vi "Intrinsic Imager.vi"() -> ()   [LabVIEW 2016]
uses:
  <vilib>/vision/Image Controls.llb/IMAQ Image.ctl
  <vilib>/userdefined/High Color/IMAQdx.ctl
  <instrlib>/niHWS/nihws.llb/niHWS Open File Permissions ID.ctl
  <vilib>/Utility/error.llb/DialogType.ctl
  <vilib>/DAQmx/read.llb/DAQmx Read (Analog Wfm 1Chan NSamp).vi
  <vilib>/Analysis/baseanly.llb/Mean (DBL).vi
  <instrlib>/niHWS/nihws.llb/niHWS Write Analog DBL.vi
  <vilib>/DAQmx/miscellaneous.llb/DAQmx Fill In Error Info.vi
  <instrlib>/niHWS/nihws.llb/niHWS Write Analog WDT.vi
  <instrlib>/niHWS/nihws.llb/niHWS Write Digital 2D U16.vi
  <vilib>/vision/NI_Vision_Development_Module.lvlib
  <resource>/objmgr/daqmx.rc
  <vilib>/Analysis/NI_AALBase.lvlib
  <vilib>/vision/driver/NI_Vision_Acquisition_Software.lvlib
panel:
  in  "Single trial":bool
  in  "Analysis":enum32{"Amp", "Angle", "Amp/Angle"}(radio)
  in  "Analyze":bool
  in  "Period (ms)":dbl=16641.0
  in  "Pixel Thr":dbl=4095.0
  in  "Magnify":bool
  in  "PseudoColor":bool
  out "Frames":u32 caption="Image Number"
  out "Rep. Fps":dbl caption="Frame Rate"
  out "Fps":dbl
  out "Ephys Rate":dbl=1000.0
  in  "Final res.":dbl=512.0
  out "Image Parameters : Bits per Pixel":u32
  out "Numeric":i32
  out "Setup":i32
  out "PPhocus?":bool
  out "file handle out":u32
  out "Recording":bool
  in  "stop":bool
  out "Raw Image":T1(plugin-control)
  out "Rec Time":dbl
  out "Photodiode display":waveform(dbl)(graph)
  in  "Recording Path":path
  in  "Rec":bool
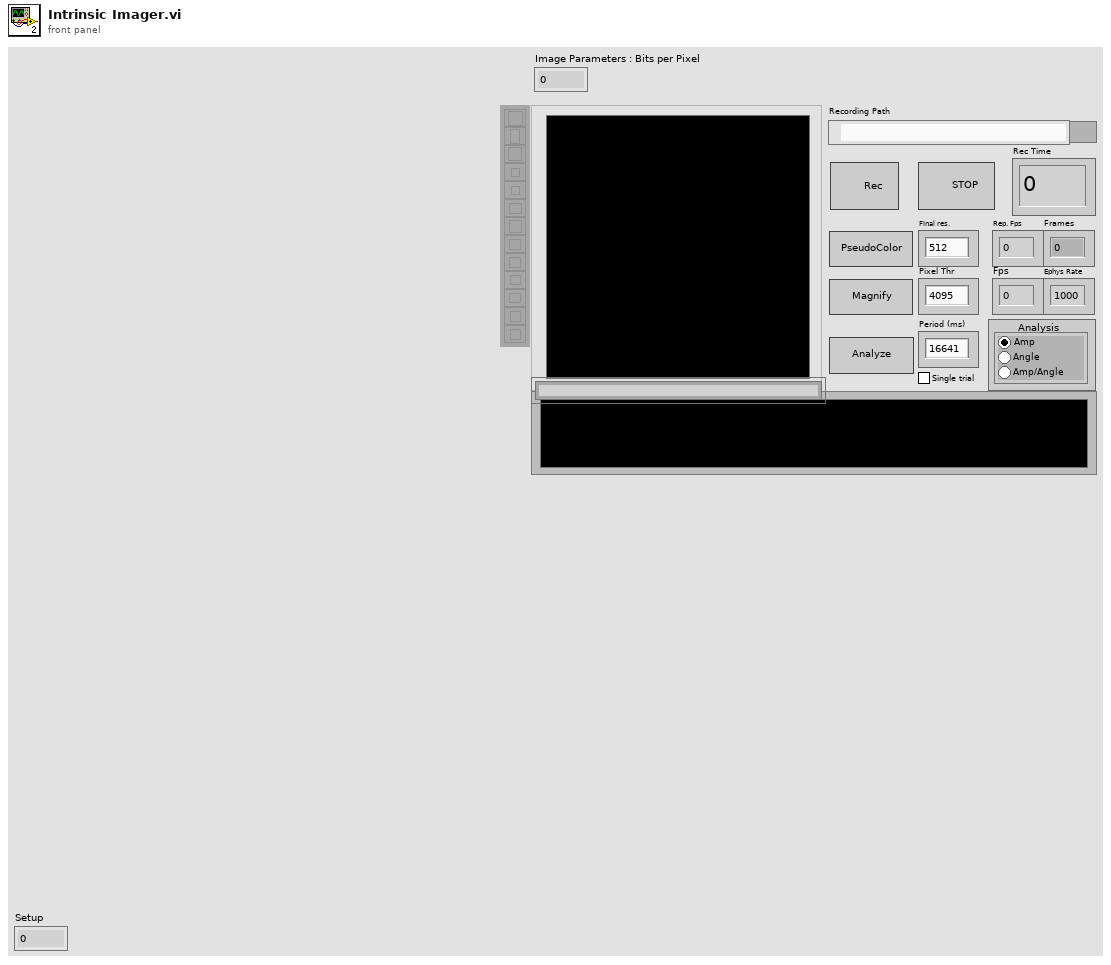
[diagram p1: front panel]
types:
  T1 = typedef "IMAQ Image.ctl" = refnum<image>
  T2 = typedef "IMAQdx.ctl" = refnum<k21>
  T3 = typedef "Image Type" = u32
  T4 = cluster{"IMAQ Session Out":refnum<k11>, "OriginalImage":T1, "error out":errorcluster, "size":cluster{dbl, i32}[], "Cropped Image":T1, "IMAQdx Session":T2, "Camera":string, "Image Type":T3, "Mirrored Image":T1, "Rotated Image":T1}
  T5 = typedef "niHWS Open File Permissions ID.ctl" = enum32{"Read Only", "Read/Write Existing", "Read/Write/Create New", "Read/Write/Create New Always"}
  T6 = enum32{"Average", "Min", "Max", "Clear  if < ", "Clear  if < or =", "Clear  if =", "Clear  if > or =", "Clear  if >"}
  T7 = enum32{"Invalid", "Standard", "Closed", "Hidden", "Minimized", "Maximized"}
  T8 = cluster{"Interpolation Type":enum32{"Zero Order", "Bilinear", "Quadratic", "Cubic", "Bilinear Fixed"}, "Destination Width":u32, "Destination Height":u32, "Fill Value":sgl}
  T9 = cluster{"Type":u32, "Version":u32, "Flags":u32, "SerialNumberHigh":u32, "SerialNumberLow":u32, "BusType":u32, "InterfaceName":string, "VendorName":string, "ModelName":string, "CameraFileName":string, "CameraAttributeURL":string}[]
  T10 = cluster{"Type":u32, "Version":u32, "Flags":u32, "SerialNumberHigh":u32, "SerialNumberLow":u32, "BusType":u32, "InterfaceName":string, "VendorName":string, "ModelName":string, "CameraFileName":string, "CameraAttributeURL":string}
  T11 = typedef "DialogType.ctl" = u16
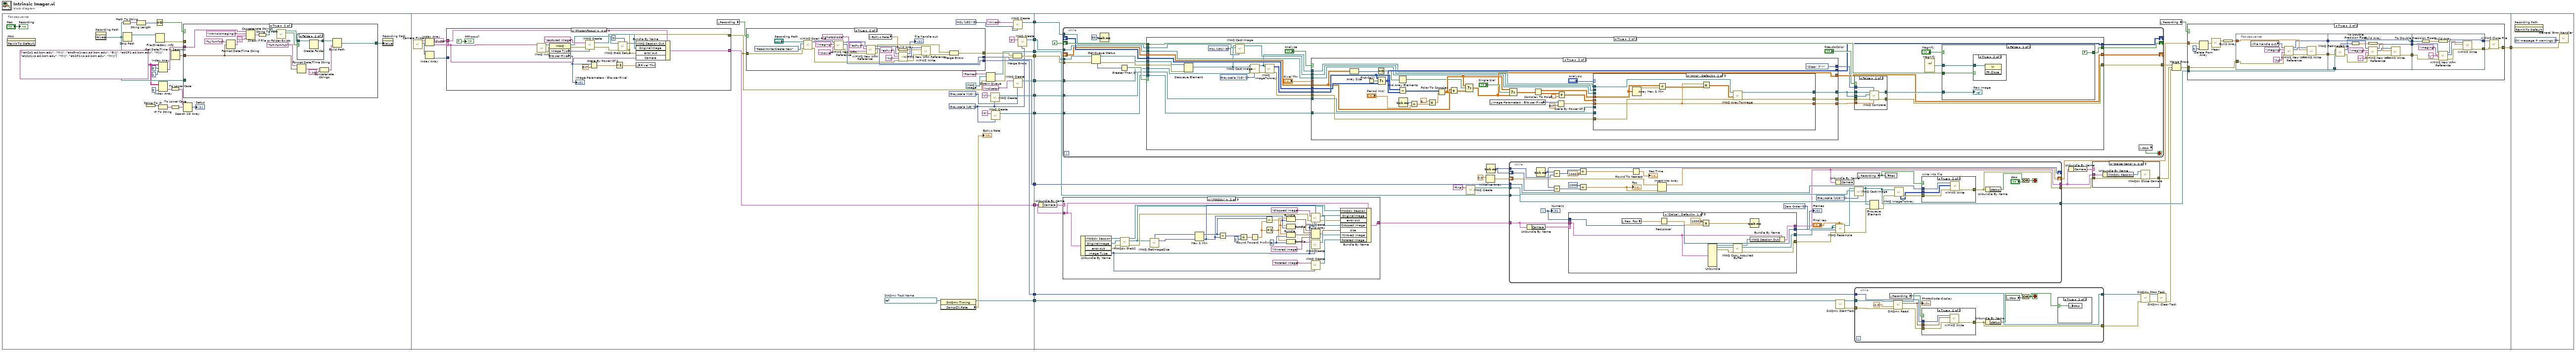
[diagram p0: block diagram]
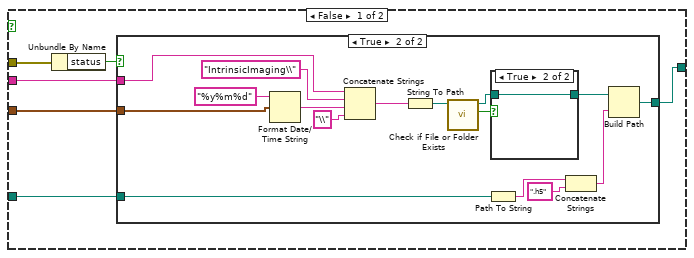
[diagram p2: hidden frame]
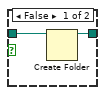
[diagram p4: hidden frame]
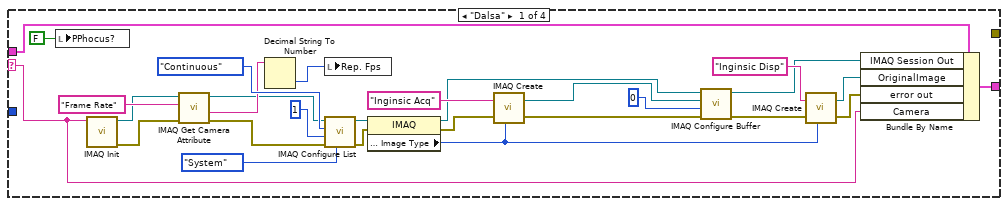
[diagram p6: hidden frame]
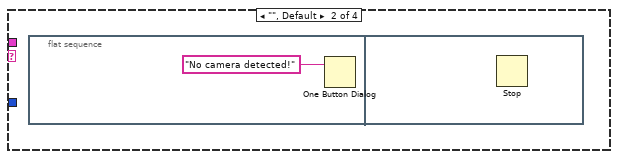
[diagram p7: hidden frame]
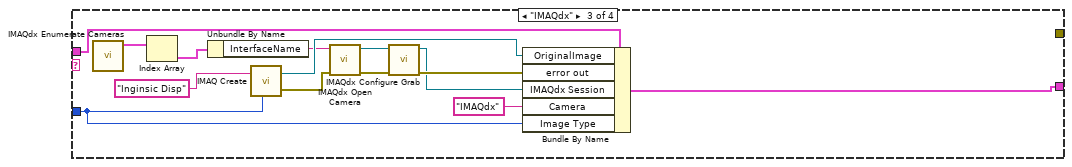
[diagram p8: hidden frame]
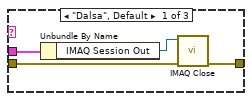
[diagram p10: hidden frame]
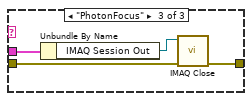
[diagram p11: hidden frame]
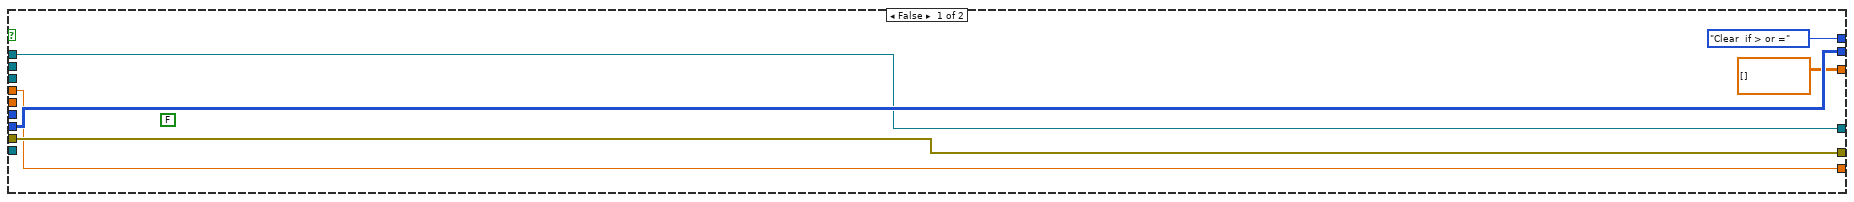
[diagram p13: hidden frame]
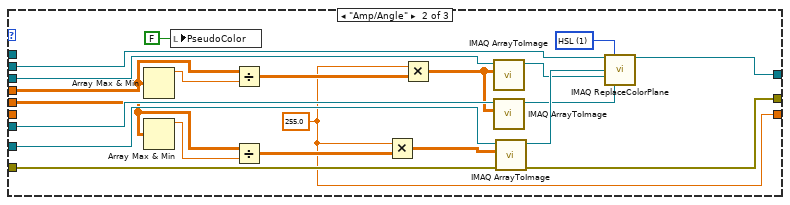
[diagram p14: hidden frame]
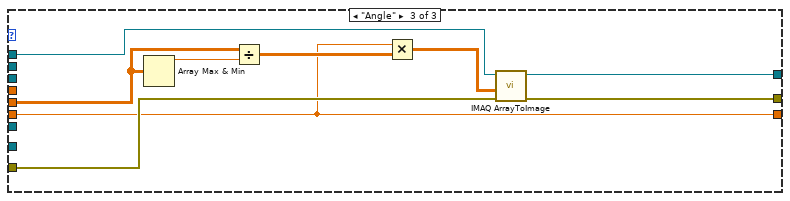
[diagram p15: hidden frame]
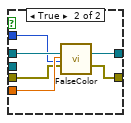
[diagram p16: hidden frame]
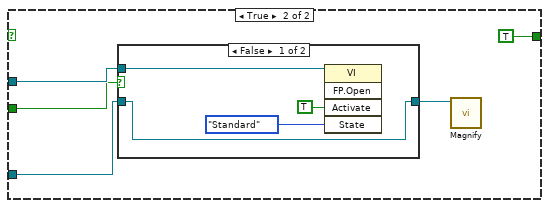
[diagram p18: hidden frame]
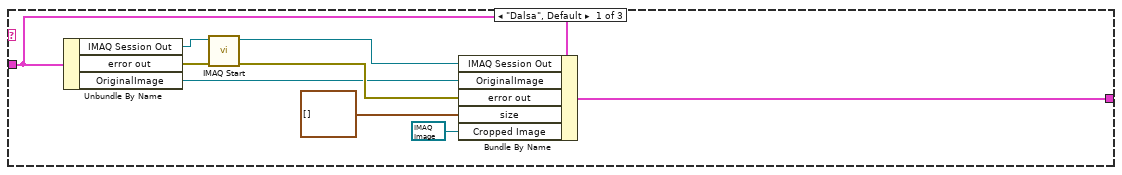
[diagram p20: hidden frame]
diagram:
  n1 = flat-sequence {
    tunnel: [w109] -> w12
    tunnel: [w108] -> w11
    tunnel: [w104] -> w9
    tunnel: [w96] -> w8
    tunnel: [w95] -> w7
    tunnel: [w92] -> w6
    tunnel: [w90] -> w5
    tunnel: [w88] -> w4
    tunnel: [w87] -> w3
    tunnel: [w83] -> w2
    tunnel: [w80] -> w1
    tunnel: w12 -> [w225]
    tunnel: w11 -> [w226]
    tunnel: [w224] -> w10
    tunnel: w9 -> [w211]
    tunnel: w8 -> [w208]
    tunnel: w7 -> [w209]
    tunnel: w6 -> [w206]
    tunnel: w5 -> [w205]
    tunnel: w4 -> [w204]
    tunnel: w3 -> [w203]
    tunnel: w2 -> [w202]
    tunnel: w1 -> [w201]
    tunnel: w10 -> [w637]
    frame #0 {
      w19 = string[][] [["at-2p1.ad.bcm.edu", "M:\\"], ["at-s5no1new.ad.bcm.edu", "E:\\"], ["at-2P1.ad.bcm.edu", "M:\\"], ["at-2p1xp.ad.bcm.edu", "M:\\"], ["at-2P1xp.ad.bcm.edu", "M:\\"]]
      n2 = invoke on="stop" class="Bool (strict)" method="Reinit To Default"() -> ()  [unwired: 3 in, 3 out]
      n3 = property on="Recording Path" class="Path"() -> ("Value"=w26:path)  [unwired: 2 in, 2 out]
      n4 = Path To String(path=w26) -> (string=w31:string)
      n5 = Strip Path(path=w26) -> (stripped path=w25:path)  [unwired: 1 out]
      n6 = String Length(string=w31) -> (length=w30:i32)
      n7 = String To IP() -> (0:w23:u32)  [unwired: 1 in]
      n8 = Equal To 0?(x=w30) -> (x = 0?=w29:bool)
      n9 = File/Directory Info(path=w25) -> (error out=w24:errorcluster)  [unwired: 1 in, 6 out]
      n10 = IP To String(2:w23) -> (0:w15:string)  [unwired: 1 in]
      n11 = Index Array(array=w19, index (row)=0 ("disabled index (row)"), index (col)=1 ("disabled index (col)")) -> (element=w18:string)
      n12 = Index Array(array=w19, index (col)=0 ("disabled index (col)")) -> (element=w17:string[])  [unwired: 1 in]
      n13 = To Lower Case(string=w17) -> (all lower case string=w16:string[])
      n14 = To Lower Case(string=w15) -> (all lower case string=w14:string)
      n15 = Get Date/Time In Seconds() -> (seconds since 1Jan1904=w32:timestamp)
      n16 = case shown="True" w29 {
        tunnel: w32 -> [w36 w65]
        tunnel: w26 -> [w37 _]
        tunnel: [w38 w63] -> w28
        tunnel: w24 -> [w34 _]
        tunnel: w18 -> [w33 w59]
        frame False {
          n17 = Unbundle By Name(w34) -> ("status"=w35:bool)
          n18 = case shown="True" w35 {
            tunnel: [w39 w46] -> w38
            tunnel: w37 -> [w39 w45]
            tunnel: w36 -> [_ w41]
            tunnel: w33 -> [_ w40]
            frame False {
            }
            frame True {
              n19 = Format Date/Time String(time format string (%c)="%y%m%d", seconds (now)=w41) -> (date/time string=w50:string)  [unwired: 1 in]
              n20 = Concatenate Strings(w40, "IntrinsicImaging\\", w50, "\\") -> (w49:string)
              n21 = String To Path(string=w49) -> (path=w55:path)
              n22 = call <vilib>:"Check if File or Folder Exists.vi"("path"=w55) -> ("file or folder exists?"=w53:bool, "dup path"=w52:path)  [unwired: 8 in, 1 out]
              n23 = Path To String(path=w45) -> (string=w42:string)
              n24 = case shown="True" w53 {
                tunnel: [w57 w58] -> w54
                tunnel: w52 -> [w56 w58]
                frame False {
                  n25 = Create Folder(path (use dialog)=w56) -> (created path=w57:path)  [unwired: 2 in, 2 out]
                }
                frame True {
                }
              }
              n26 = Concatenate Strings(w42, ".h5" ("string")) -> (w43:string)
              n27 = Build Path(base path=w54, name or relative path=w43) -> (appended path=w46:path)
            }
          }
        }
        frame True {
          n28 = Format Date/Time String(time format string (%c)="%y%m%d", seconds (now)=w65) -> (date/time string=w71:string)  [unwired: 1 in]
          n29 = Concatenate Strings(w59, "IntrinsicImaging\\", w71, "\\") -> (w72:string)
          n30 = String To Path(string=w72) -> (path=w64:path)
          n31 = call <vilib>:"Check if File or Folder Exists.vi"("path"=w64) -> ("file or folder exists?"=w68:bool, "dup path"=w69:path)  [unwired: 8 in, 1 out]
          n32 = case shown="False" w68 {
            tunnel: [w76 w77] -> w67
            tunnel: w69 -> [w75 w77]
            frame False {
              n33 = Create Folder(path (use dialog)=w75) -> (created path=w76:path)  [unwired: 2 in, 2 out]
            }
            frame True {
            }
          }
          n34 = Format Date/Time String(time format string (%c)="%H-%M-%S", seconds (now)=w65) -> (date/time string=w62:string)  [unwired: 1 in]
          n35 = Concatenate Strings(w62, ".h5" ("string")) -> (w60:string)
          n36 = Build Path(base path=w67, name or relative path=w60) -> (appended path=w63:path)
        }
      }
      n37 = Search 1D Array(1D array=w16, element=w14) -> (index of element=→"Setup":i32)  [unwired: 1 in]
      n38 = property on="Recording Path" class="Path"("Value"=w28) -> ()  [unwired: 2 in, 2 out]
      "Recording" <- "Rec"
    }
    frame #1 {
      w84 = T3 1 items=["Grayscale (U8)", "Grayscale (I16)", "Grayscale (SGL)", "Complex (CSG)", "RGB (U32)", "HSL (U32)", "RGB (U64)", "Grayscale (U16)"] ("Image Type")
      w86 = T3 0 items=["Grayscale (U8)", "Grayscale (I16)", "Grayscale (SGL)", "Complex (CSG)", "RGB (U32)", "HSL (U32)", "RGB (U64)", "Grayscale (U16)"] ("Image Type")
      w93 = T3 5 items=["Grayscale (U8)", "Grayscale (I16)", "Grayscale (SGL)", "Complex (CSG)", "RGB (U32)", "HSL (U32)", "RGB (U64)", "Grayscale (U16)"] ("Image Type")
      w106 = refnum<k21> "Photodiode Intrinsic Imaging"  # DAQmx Task Name
      n39 = call "Camera Finder.vi"() -> ("Image type"=w79:T3[], "IMAQ Interfaces"=w102:string[])  [unwired: 10 in]
      n40 = Index Array(array=w102) -> (element=w103:string)  [unwired: 1 in]
      n41 = Index Array(array=w79) -> (element=w78:T3)  [unwired: 1 in]
      n42 = case shown="\"PhotonFocus\"" w103 {
        selector: w103 -> [w110 _ _ w153]
        tunnel: [_ _ _ w155] -> w99
        tunnel: [w111 _ w149 w154] -> w80
        tunnel: T4 {"IMAQ Session Out"=refnum, "OriginalImage"=refnum, "error out"={"status"=FALSE, "code"=0, "source"=""}, "size"=[], "Cropped Image"=refnum, "IMAQdx Session"="", "Camera"="", "Image Type"=0, "Mirrored Image"=refnum, "Rotated Image"=refnum} ("cluster") -> [w115 _ w148 w158]
        tunnel: w78 -> [_ _ w143 _]
        frame "Dalsa" {
          n43 = local write "PPhocus?"(FALSE ("PPhocus?")) -> ()
          n44 = call <vilib>:"IMAQ Init.vi"("Interface Name"=w110) -> ("error out"=w120:errorcluster, "IMAQ Session Out"=w121:refnum<k11>)  [unwired: 9 in]
          n45 = call <vilib>:"IMAQ Get Camera Attribute.vi"("error in (no error)"=w120, "Camera Attribute"="Frame Rate", "IMAQ Session In"=w121) -> ("error out"=w116:errorcluster, "Attribute Value"=w118:string, "IMAQ Session Out"=w117:refnum<k11>)  [unwired: 4 in]
          n46 = Decimal String To Number(string=w118) -> (number=w119:i32)  [unwired: 2 in, 1 out]
          n47 = local write "Rep. Fps"(w119) -> ()
          n48 = call <vilib>:"IMAQ Configure List.vi"("Memory Location"=enum16{"System", "Onboard"}."System", "error in (no error)"=w116, "Number of buffers"=u32 1, "Continuous?"=enum16{"One-Shot", "Continuous"}."Continuous" ("Continuous ?"), "IMAQ Session In"=w117) -> ("error out"=w129:errorcluster, "IMAQ Session Out"=w130:refnum<k11>)  [unwired: 5 in]
          n49 = property class="IMAQ"(reference=w130, error in=w129) -> (reference out=w128:refnum<k11>, error out=w127:errorcluster, "Image Parameters : Image Type"=w126:u32)
          n50 = call "IMAQ Create"("Image Name"="Inginsic Acq", "Image Type"=w126, "error in (no error)"=w127) -> ("New Image"=w123:T1, "error out"=w133:errorcluster)  [unwired: 2 in]
          n51 = call <vilib>:"IMAQ Configure Buffer.vi"("error in (no error)"=w133, "Buffer Number"=u32 0, "Image In"=w123, "IMAQ Session In"=w128) -> ("error out"=w125:errorcluster, "IMAQ Session Out"=w114:refnum<k11>)  [unwired: 6 in]
          n52 = call "IMAQ Create"("Image Name"="Inginsic Disp", "Image Type"=w126, "error in (no error)"=w125) -> ("New Image"=w113:T1, "error out"=w112:errorcluster)  [unwired: 2 in]
          n53 = Bundle By Name(cluster=w115, "IMAQ Session Out"=w114, "OriginalImage"=w113, "error out"=w112, "Camera"=w110) -> (w111:T4)
        }
        frame "", Default {
          n54 = flat-sequence {
            frame #0 {
              n55 = One Button Dialog(message="No camera detected!" ("error source (\" \")")) -> ()  [unwired: 1 in, 1 out]
            }
            frame #1 {
              n56 = Stop() -> ()  [unwired: 1 in]
            }
          }
        }
        frame "IMAQdx" {
          n57 = call <vilib>:"IMAQdx Enumerate Cameras.vi"() -> ("Camera Information Array"=w142:T9)  [unwired: 10 in, 1 out]
          n58 = Index Array(array=w142) -> (element=w141:T10)  [unwired: 1 in]
          n59 = Unbundle By Name(w141) -> ("InterfaceName"=w140:string)
          n60 = call "IMAQ Create"("Image Name"="Inginsic Disp", "Image Type"=w143) -> ("New Image"=w151:T1, "error out"=w150:errorcluster)  [unwired: 3 in]
          n61 = call <vilib>:"IMAQdx Open Camera.vi"("error in"=w150, "Session In"=w140) -> ("error out"=w146:errorcluster, "Session Out"=w147:T2)  [unwired: 8 in]
          n62 = call <vilib>:"IMAQdx Configure Grab.vi"("error in"=w146, "Session In"=w147) -> ("error out"=w145:errorcluster, "Session Out"=w144:T2)  [unwired: 8 in]
          n63 = Bundle By Name(cluster=w148, "OriginalImage"=w151, "error out"=w145, "IMAQdx Session"=w144, "Camera"="IMAQdx", "Image Type"=w143) -> (w149:T4)
        }
        frame "PhotonFocus" {
          n64 = call <vilib>:"IMAQ Init.vi"("Interface Name"=w153) -> ("error out"=w170:errorcluster, "IMAQ Session Out"=w169:refnum<k11>)  [unwired: 1 in, 8 out]
          n65 = property class="IMAQ"(reference=w169, error in=w170) -> (reference out=w164:refnum<k11>, error out=w167:errorcluster, "Image Parameters : Image Type"=w168:u32, "Bits per Pixel"=w162:u32)
          "Image Parameters : Bits per Pixel" <- w162
          n66 = call "IMAQ Create"("Image Name"="captured image", "Image Type"=w168, "error in (no error)"=w167) -> ("New Image"=w157:T1, "error out"=w165:errorcluster)  [unwired: 1 in, 1 out]
          n67 = Scale By Power Of 2(n=w162, x=ext 1.0) -> (x*2^n=w160:ext)
          n68 = Decrement(x=w160) -> (x-1=w159:ext)
          n69 = call <vilib>:"IMAQ Grab Setup.vi"("Channel"=0, "error in (no error)"=w165, "IMAQ Session In"=w164) -> ("error out"=w155:errorcluster, "IMAQ Session Out"=w156:refnum<k11>)  [unwired: 7 out]
          n70 = Bundle By Name(cluster=w158, "IMAQ Session Out"=w156, "OriginalImage"=w157, "error out"=w155, "Camera"=w153) -> (w154:T4)
          n71 = local write "Pixel Thr"(w159) -> ()
          "PPhocus?" <- TRUE ("PPhocus?")
        }
      }
      n72 = local read "Recording"() -> (w107:bool)
      n73 = case shown="True" w107 {
        tunnel: [_ w195] -> w109
        tunnel: [_ w175] -> w98
        tunnel: [_ w193] -> w108
        tunnel: w99 -> [_ w172]
        frame False {
        }
        frame True {
          n74 = call <instrlib>:"niHWS Open File.vi"("error in (no error)"=w172, "permissions (0:read only)"=niHWS_Open_File_Permissions_ID."Read/Write/Create New", "file path"="Recording Path") -> ("error out"=w190:errorcluster, "file handle"=w182:u32)  [unwired: 7 in]
          n75 = call <instrlib>:"niHWS New Wfm Reference.vi"("waveform name (empty)"="movie" ("format string"), "group name (empty)"="imaging", "file handle in"=w182) -> ("error out"=w178:errorcluster, "waveform reference"=w195:u32, "file handle out"=w179:u32)  [unwired: 6 in]
          n76 = call <instrlib>:"niHWS New Wfm Reference.vi"("error in (no error)"=w178, "waveform name (empty)"="photodiode", "group name (empty)"="ephys", "file handle in"=w179) -> ("error out"=w177:errorcluster, "waveform reference"=w193:u32, "file handle out"=w194:u32)  [unwired: 5 in]
          n77 = local read "Ephys Rate"() -> (w173:dbl)
          n78 = Build Array(w173) -> (w186:dbl[])
          n79 = call <instrlib>:"niHWS New Wfm Reference.vi"("error in (no error)"=w190, "waveform name (empty)"="hz" ("group name (empty)"), "group name (empty)"="ephys", "file handle in"=w194) -> ("error out"=w185:errorcluster, "waveform reference"=w189:u32, "file handle out"=→"file handle out":u32)  [unwired: 5 in]
          n80 = call-poly <instrlib>:"niHWS Write.vi"("error in (no error)"=w185, "data"=w186, "waveform reference in"=w189) -> ("error out"=w176:errorcluster)  [unwired: 7 in, 1 out]
          n81 = Merge Errors(w177, w176) -> (w175:errorcluster)
        }
      }
      n82 = property class="DAQmx Timing"(reference=w106) -> (reference out=w104:refnum<k21>, "SampClk.Rate"=→"Ephys Rate":dbl)  [unwired: 1 in, 1 out]
      n83 = Obtain Queue(name (unnamed)="Frames", element data type=T1 refnum ("New Image"), error in (no error)=w99) -> (queue out=w95:refnum<queue>, error out=w97:errorcluster)  [unwired: 2 in, 1 out]
      n84 = call "IMAQ Create"("Image Name"="V", "Image Type"=w86) -> ("New Image"=w90:T1)  [unwired: 3 in, 1 out]
      n85 = call "IMAQ Create"("Image Name"="H", "Image Type"=w86) -> ("New Image"=w88:T1)  [unwired: 3 in, 1 out]
      n86 = Merge Errors(w98, w97) -> (w96:errorcluster)
      n87 = call "IMAQ Create"("Image Name"="mixed", "Image Type"=w93) -> ("New Image"=w92:T1)  [unwired: 3 in, 1 out]
      n88 = call "IMAQ Create"("Image Name"="Indicator", "Image Type"=w84) -> ("New Image"=w83:T1)  [unwired: 3 in, 1 out]
      n89 = call "IMAQ Create"("Image Name"="S", "Image Type"=w86) -> ("New Image"=w87:T1)  [unwired: 3 in, 1 out]
    }
    frame #2 {
      n90 = Unbundle By Name(w201) -> ("Camera"=w200:string)
      n91 = while {
        shift-right: [w262] -> _
        shift-left: FALSE -> [w261]
        tunnel: w209 -> [w259]
        tunnel: w208 -> [w255]
        tunnel: [w253] -> w207
        shift-right: [w252] -> _
        shift-left: _ -> [w251]
        shift-right: [w250] -> _
        shift-left: _ -> [w249]
        tunnel: w206 -> [w248]
        tunnel: w205 -> [w247]
        tunnel: w204 -> [w246]
        tunnel: w203 -> [w245]
        tunnel: w202 -> [w244]
        stop <- w263 stop-if-true
        n92 = Get Queue Status(queue=w259, error in (no error)=w255) -> (queue out=w256:refnum<queue>, error out=w254:errorcluster, # elements in queue=w258:i32)  [unwired: 1 in, 5 out]
        n93 = Wait (ms)(milliseconds to wait=u32 50) -> ()  [unwired: 1 out]
        n94 = Greater Than 0?(x=w258) -> (x > 0?=w257:bool)
        n95 = case shown="True" w257 {
          tunnel: [w267 w297] -> w262
          tunnel: w261 -> [w267 w296]
          tunnel: w256 -> [_ w293]
          tunnel: w254 -> [w266 w292]
          tunnel: [w266 w290] -> w253
          tunnel: [w265 w288] -> w252
          tunnel: w251 -> [w265 w287]
          tunnel: [w264 w286] -> w250
          tunnel: w249 -> [w264 w285]
          tunnel: w248 -> [_ w272]
          tunnel: w247 -> [_ w271]
          tunnel: w246 -> [_ w270]
          tunnel: w245 -> [_ w269]
          tunnel: w244 -> [_ w268]
          frame False {
          }
          frame True {
            w274 = T3 5 items=["Grayscale (U8)", "Grayscale (I16)", "Grayscale (SGL)", "Complex (CSG)", "RGB (U32)", "HSL (U32)", "RGB (U64)", "Grayscale (U16)"] ("Image Type")
            w276 = T3 1 items=["Grayscale (U8)", "Grayscale (I16)", "Grayscale (SGL)", "Complex (CSG)", "RGB (U32)", "HSL (U32)", "RGB (U64)", "Grayscale (U16)"] ("Image Type")
            n96 = Dequeue Element(queue=w293, error in (no error)=w292) -> (element=w275:T1)  [unwired: 1 in, 3 out]
            n97 = call "IMAQ Cast Image"("Image Type"=w274, "Image Dst"=w272, "Image Src"=w275) -> ("Image Dst Out"=w273:T1)  [unwired: 7 in, 1 out]
            n98 = call "IMAQ Cast Image"("Image Type"=w276, "Image Dst"=w268, "Image Src"=w275) -> ("error out"=w282:errorcluster, "Image Dst Out"=w284:T1)  [unwired: 7 in]
            n99 = call "IMAQ ImageToArray"("error in (no error)"=w282, "Image"=w284) -> ("error out"=w281:errorcluster, "Image Pixels (I16)"=w289:i16[][])  [unwired: 2 in, 3 out]
            n100 = case shown="True" "Analyze" {
              tunnel: w289 -> [w305 w340]
              tunnel: [w305 w339] -> w288
              tunnel: w287 -> [_ w341]
              tunnel: [cdb[][] [] w310] -> w286
              tunnel: w285 -> [_ w314]
              tunnel: w284 -> [w304 w329]
              tunnel: [w304 w328] -> w283
              tunnel: w281 -> [w303 w326]
              tunnel: [w303 w327] -> w280
              tunnel: [w302 w320] -> w279
              tunnel: "Pixel Thr" -> [w302 _]
              tunnel: [T6."Clear  if > or =" ("Operator") T6."Clear  if >" ("Operator")] -> w277
              tunnel: w273 -> [_ w309]
              tunnel: w270 -> [_ w308]
              tunnel: w269 -> [_ w307]
              tunnel: w271 -> [_ w306]
              frame False {
                (unwired) FALSE
              }
              frame True {
                n101 = Array Size(array=w314) -> (size(s)=w313:i32[])
                n102 = First Call?() -> (First Call?: T/F=w342:bool)
                n103 = Equal To 0?(x=w313) -> (x = 0?=w312:bool[])
                n104 = Select(t=w340, s=w342, f=w341) -> (s? t:f=w339:i16[][])
                n105 = And Array Elements(Boolean array=w312) -> (logical AND=w311:bool)
                n106 = Subtract(x=w340, y=w339) -> (x-y=w333:i16[][])
                n107 = Tick Count (ms)() -> (millisecond timer value=w336:u32)
                n108 = Divide(x=w336, y="Period (ms)") -> (x/y=w334:dbl)
                n109 = Multiply(x=6.283185307179586, y=w334) -> (x*y=w338:dbl)
                n110 = Polar To Complex(1:w338, 2:w333) -> (0:w315:cdb[][])
                n111 = Add(x=w314, y=w315) -> (x+y=w316:cdb[][])
                n112 = Select(t=w315, s=w311, f=w316) -> (s? t:f=w310:cdb[][])
                n113 = local read "Image Parameters : Bits per Pixel"() -> (w322:u32)
                n114 = Select(t=w315, s="Single trial", f=w310) -> (s? t:f=w317:cdb[][])
                n115 = Complex To Polar(r * e^(i*theta)=w317) -> (r=w325:dbl[][], theta=w332:dbl[][])
                n116 = Scale By Power Of 2(n=w322, x=ext 1.0) -> (x*2^n=w321:ext)
                n117 = Add(x=w332, y=3.141592653589793) -> (x+y=w324:dbl[][])
                n118 = case shown="\"Amp\", Default" "Analysis" {
                  tunnel: w329 -> [w343 _ w378]
                  tunnel: [w349 w364 w375] -> w328
                  tunnel: [w348 w367 w376] -> w327
                  tunnel: w326 -> [w347 w368 w377]
                  tunnel: w325 -> [w346 w352 _]
                  tunnel: w324 -> [_ w353 w379]
                  tunnel: w321 -> [w345 _ w374]
                  tunnel: [w345 w354 w374] -> w320
                  tunnel: w309 -> [_ w365 _]
                  tunnel: w308 -> [_ w360 _]
                  tunnel: w307 -> [_ w359 _]
                  tunnel: w306 -> [_ w357 _]
                  frame "Amp", Default {
                    n119 = Array Max & Min(array=w346) -> (max value=w350:dbl)  [unwired: 3 out]
                    n120 = Divide(x=w346, y=w350) -> (x/y=w351:dbl[][])
                    n121 = Multiply(x=w345, y=w351) -> (x*y=w344:ext[][])
                    n122 = call "IMAQ ArrayToImage"("error in (no error)"=w347, "Image Pixels (I16)"=w344, "Image"=w343) -> ("error out"=w348:errorcluster, "Image Out"=w349:T1)  [unwired: 7 in]
                  }
                  frame "Amp/Angle" {
                    w366 = u16 1 items=["RGB", "HSL", "HSV", "HSI"] ("Color Mode")
                    w354 = 255.0
                    n123 = Array Max & Min(array=w352) -> (max value=w370:dbl)  [unwired: 3 out]
                    n124 = Array Max & Min(array=w353) -> (max value=w371:dbl)  [unwired: 3 out]
                    n125 = local write "PseudoColor"(FALSE ("PseudoColor")) -> ()
                    n126 = Divide(x=w352, y=w370) -> (x/y=w369:dbl[][])
                    n127 = Divide(x=w353, y=w371) -> (x/y=w372:dbl[][])
                    n128 = Multiply(x=w354, y=w372) -> (x*y=w362:dbl[][])
                    n129 = Multiply(x=w354, y=w369) -> (x*y=w356:dbl[][])
                    n130 = call "IMAQ ArrayToImage"("Image Pixels (U8)"=w356, "Image"=w359) -> ("Image Out"=w358:T1)  [unwired: 8 in, 1 out]
                    n131 = call "IMAQ ArrayToImage"("Image Pixels (U8)"=w356, "Image"=w357) -> ("Image Out"=w355:T1)  [unwired: 8 in, 1 out]
                    n132 = call "IMAQ ArrayToImage"("error in (no error)"=w368, "Image Pixels (U8)"=w362, "Image"=w360) -> ("error out"=w367:errorcluster, "Image Out"=w361:T1)  [unwired: 7 in]
                    n133 = call "IMAQ ReplaceColorPlane"("Image Src"=w365, "Color Mode"=w366, "Red or Hue Plane"=w361, "Green or Sat Plane"=w358, "Blue or Luma or Val or Inten Plane"=w355) -> ("Image Dst Out"=w364:T1)  [unwired: 9 in, 1 out]
                  }
                  frame "Angle" {
                    n134 = Array Max & Min(array=w379) -> (max value=w380:dbl)  [unwired: 3 out]
                    n135 = Divide(x=w379, y=w380) -> (x/y=w381:dbl[][])
                    n136 = Multiply(x=w374, y=w381) -> (x*y=w373:ext[][])
                    n137 = call "IMAQ ArrayToImage"("error in (no error)"=w377, "Image Pixels (I16)"=w373, "Image"=w378) -> ("error out"=w376:errorcluster, "Image Out"=w375:T1)  [unwired: 7 in]
                  }
                }
              }
            }
            n138 = case shown="False" "PseudoColor" {
              tunnel: w283 -> [w388 w394]
              tunnel: w283 -> [w387 _]
              tunnel: w277 -> [w386 w389]
              tunnel: w279 -> [w385 w392]
              tunnel: [w384 w393] -> w295
              tunnel: w280 -> [w383 w391]
              tunnel: [w382 w390] -> w290
              frame False {
                n139 = call "IMAQ Compare"("Constant"=w385, "Operator"=w386, "error in (no error)"=w383, "Image Dst"=w387, "Image Src A"=w388) -> ("error out"=w382:errorcluster, "Image Dst Out"=w384:T1)  [unwired: 5 in]
              }
              frame True {
                n140 = call "FalseColor.vi"("Image"=w394, "maxValue"=w392, "Operator"=w389, "error in (no error)"=w391) -> ("Image Dst Out"=w393:T1, "error out"=w390:errorcluster)  [unwired: 22 in]
              }
            }
            n141 = vi-ref "Magnify.vi"() -> (w299:refnum<vi>)
            n142 = case shown="False" "Magnify" {
              tunnel: w299 -> [w398 w404]
              tunnel: [FALSE TRUE] -> w297
              tunnel: w296 -> [w397 w402]
              tunnel: w295 -> [w395 w401]
              frame False {
                n143 = case shown="True" w397 {
                  tunnel: w398 -> [_ w399]
                  frame False {
                  }
                  frame True {
                    n144 = invoke class="VI" method="FP.Close"(reference=w399) -> ()  [unwired: 2 in, 3 out]
                  }
                }
                "Raw Image" <- w395
              }
              frame True {
                n145 = case shown="False" w402 {
                  tunnel: w404 -> [w407 _]
                  tunnel: w401 -> [w405 w409]
                  tunnel: [w405 w409] -> w400
                  frame False {
                    n146 = invoke class="VI" method="FP.Open"(reference=w407, "Activate"=TRUE ("Wait Until Done"), "State"=T7."Standard") -> ()  [unwired: 2 in, 5 out]
                  }
                  frame True {
                  }
                }
                n147 = call "Magnify.vi"("Camera 2"=w400) -> ()  [unwired: 11 in]
              }
            }
          }
        }
        n148 = local read "stop"() -> (w263:bool)
      }
      n149 = case shown="\"IMAQdx\"" w200 {
        tunnel: [w413 w425 w453] -> w212
        tunnel: w201 -> [w418 w431 w459]
        frame "Dalsa", Default {
          n150 = Unbundle By Name(w418) -> ("IMAQ Session Out"=w412:refnum<k11>, "error out"=w411:errorcluster, "OriginalImage"=w410:T1)
          n151 = call <vilib>:"IMAQ Start.vi"("error in (no error)"=w411, "IMAQ Session In"=w412) -> ("error out"=w416:errorcluster, "IMAQ Session Out"=w417:refnum<k11>)  [unwired: 8 in]
          n152 = Bundle By Name(cluster=w418, "IMAQ Session Out"=w417, "OriginalImage"=w410, "error out"=w416, "size"=cluster{dbl, i32}[] [], "Cropped Image"=T1 refnum ("New Image")) -> (w413:T4)
        }
        frame "IMAQdx" {
          w447 = 0
          n153 = Unbundle By Name(w431) -> ("IMAQdx Session"=w434:T2, "OriginalImage"=w433:T1, "error out"=w432:errorcluster, "Image Type"=w420:T3)
          n154 = call <vilib>:"IMAQdx Grab2.vi"("error in"=w432, "Image In"=w433, "Session In"=w434) -> ("error out"=w426:errorcluster, "Image Out"=w419:T1, "Session Out"=w428:T2)  [unwired: 5 in, 1 out]
          n155 = call "IMAQ GetImageSize"("Image"=w419) -> ("Y Resolution"=w448:i32, "X Resolution"=w449:i32)  [unwired: 3 in, 1 out]
          n156 = Max & Min(x=w449, y=w448) -> (max(x,y)=w440:i32, min(x,y)=w446:i32)
          n157 = Subtract(x=w440, y=w446) -> (x-y=w445:i32)
          n158 = Divide(x=w445, y=2) -> (x/y=w443:dbl)
          n159 = Round Toward +Infinity(x=w443) -> (ceil(x): smallest int >= x=w441:dbl)
          n160 = Subtract(x=w440, y=w441) -> (x-y=w439:dbl)
          n161 = Increment(x=w441) -> (x+1=w442:dbl)
          n162 = Bundle(w442, w446) -> (w435:cluster{dbl, i32})  [unwired: 1 in]
          n163 = Bundle(w439, w446) -> (w438:cluster{dbl, i32})  [unwired: 1 in]
          n164 = Bundle(w439, w447) -> (w437:cluster{dbl, i32})  [unwired: 1 in]
          n165 = Bundle(w442, w447) -> (w436:cluster{dbl, i32})  [unwired: 1 in]
          n166 = call "IMAQ Create"("Border Size"=w446, "Image Name"="chopped image", "Image Type"=w420, "error in (no error)"=w426) -> ("New Image"=w429:T1, "error out"=w427:errorcluster)  [unwired: 1 out]
          n167 = Build Array(w435, w438, w437, w436) -> (w430:cluster{dbl, i32}[])
          n168 = call "IMAQ Create"("Image Name"="Mirrored image", "Image Type"=w420) -> ("New Image"=w422:T1)  [unwired: 2 in, 2 out]
          n169 = call "IMAQ Create"("Image Name"="Rotated image", "Image Type"=w420) -> ("New Image"=w421:T1)  [unwired: 2 in, 2 out]
          n170 = Bundle By Name(cluster=w431, "IMAQdx Session"=w428, "OriginalImage"=w419, "error out"=w427, "Cropped Image"=w429, "size"=w430, "Mirrored Image"=w422, "Rotated Image"=w421) -> (w425:T4)
        }
        frame "PhotonFocus" {
          w472 = 0
          w476 = T3 7 items=["Grayscale (U8)", "Grayscale (I16)", "Grayscale (SGL)", "Complex (CSG)", "RGB (U32)", "HSL (U32)", "RGB (U64)", "Grayscale (U16)"] ("Image Type")
          n171 = Unbundle By Name(w459) -> ("IMAQ Session Out"=w452:refnum<k11>, "OriginalImage"=w451:T1)
          n172 = call <vilib>:"IMAQ Grab Acquire.vi"("Immediate?"=TRUE, "Image In"=w451, "IMAQ Session In"=w452) -> ("error out"=w456:errorcluster, "Image Out"=w457:T1, "IMAQ Session Out"=w458:refnum<k11>)  [unwired: 1 in, 5 out]
          n173 = call "IMAQ GetImageSize"("Image"=w457) -> ("Y Resolution"=w473:i32, "X Resolution"=w474:i32)  [unwired: 3 in, 1 out]
          n174 = Max & Min(x=w474, y=w473) -> (max(x,y)=w465:i32, min(x,y)=w471:i32)
          n175 = Subtract(x=w465, y=w471) -> (x-y=w470:i32)
          n176 = Divide(x=w470, y=2) -> (x/y=w468:dbl)
          n177 = Round Toward +Infinity(x=w468) -> (ceil(x): smallest int >= x=w466:dbl)
          n178 = Subtract(x=w465, y=w466) -> (x-y=w464:dbl)
          n179 = Increment(x=w466) -> (x+1=w467:dbl)
          n180 = Bundle(w467, w471) -> (w460:cluster{dbl, i32})  [unwired: 1 in]
          n181 = Bundle(w464, w471) -> (w463:cluster{dbl, i32})  [unwired: 1 in]
          n182 = Bundle(w464, w472) -> (w462:cluster{dbl, i32})  [unwired: 1 in]
          n183 = Bundle(w467, w472) -> (w461:cluster{dbl, i32})  [unwired: 1 in]
          n184 = Build Array(w460, w463, w462, w461) -> (w455:cluster{dbl, i32}[])
          n185 = call "IMAQ Create"("Border Size"=w471, "Image Name"="chopped image", "Image Type"=w476) -> ("New Image"=w454:T1)  [unwired: 1 in, 2 out]
          n186 = Bundle By Name(cluster=w459, "IMAQ Session Out"=w458, "OriginalImage"=w457, "error out"=w456, "size"=w455, "Cropped Image"=w454) -> (w453:T4)
        }
      }
      n187 = call "IMAQ Create"("Image Name"="Final") -> ("New Image"=w196:T1)  [unwired: 4 in, 1 out]
      n188 = Initialize Array(0.0 ("element")) -> (w222:dbl[])  [unwired: 1 in]
      n189 = Tick Count (ms)() -> (millisecond timer value=w231:u32)
      n190 = while {
        tunnel: w225 -> [w581]
        shift-right: [w576] -> _
        shift-left: w231 -> [w580]
        tunnel: w231 -> [w575]
        shift-right: [w569] -> w220
        shift-left: w222 -> [w570]
        tunnel: [w565] -> w215
        tunnel: [w549] -> w217
        tunnel: w212 -> [w554]
        tunnel: w209 -> [w557]
        tunnel: [w551] -> w198
        tunnel: w196 -> [w547]
        i -> [w559]
        stop <- w566 stop-if-true
        w548 = T3 7 items=["Grayscale (U8)", "Grayscale (I16)", "Grayscale (SGL)", "Complex (CSG)", "RGB (U32)", "HSL (U32)", "RGB (U64)", "Grayscale (U16)"] ("Image Type")
        w558 = u32 0 items=["Zero Order", "Bi-Linear", "Quadratic", "Cubic Spline"] ("Interpolation Type")
        n191 = Unbundle By Name(w554) -> ("Camera"=w553:string)
        n192 = Tick Count (ms)() -> (millisecond timer value=w576:u32)
        n193 = Subtract(x=w576, y=w575) -> (x-y=w574:u32)
        n194 = Subtract(x=w576, y=w580) -> (x-y=w579:u32)
        n195 = case shown="\"Dalsa\", Default" w553 {
          tunnel: [w584 w601 w618] -> w561
          tunnel: [w594 w606 w629] -> w560
          tunnel: w559 -> [w594 _ _]
          tunnel: w554 -> [w586 w605 w620]
          tunnel: [w583 w603 w617] -> w551
          tunnel: [w582 w602 w616] -> w552
          frame "Dalsa", Default {
            n196 = local read "Rep. Fps"() -> (w590:dbl)
            n197 = Reciprocal(x=w590) -> (1/x=w589:dbl)
            n198 = Multiply(x=1000.0, y=w589) -> (x*y=w587:dbl)
            n199 = Unbundle(w586) -> ("IMAQ Session Out"=w593:refnum<k11>, "OriginalImage"=w592:T1, "error out"=w591:errorcluster)  [unwired: 7 out]
            n200 = call <vilib>:"IMAQ Copy Acquired Buffer.vi"("IMAQ Session In"=w593, "Image In"=w592, "error in (no error)"=w591) -> ("IMAQ Session Out"=w585:refnum<k11>, "Image Out"=w584:T1, "error out"=w582:errorcluster)  [unwired: 8 in, 2 out]
            n201 = Wait (ms)(milliseconds to wait=w587) -> ()  [unwired: 1 out]
            n202 = Bundle By Name(cluster=w586, "IMAQ Session Out"=w585) -> (w583:T4)
          }
          frame "IMAQdx" {
            n203 = Unbundle By Name(w605) -> ("IMAQdx Session"=w612:T2, "OriginalImage"=w611:T1, "error out"=w610:errorcluster, "Cropped Image"=w600:T1, "size"=w608:cluster{dbl, i32}[], "Rotated Image"=w598:T1)  [unwired: 1 out]
            n204 = call <vilib>:"IMAQdx Grab2.vi"("error in"=w610, "Image In"=w611, "Session In"=w612) -> ("error out"=w609:errorcluster, "Buffer Number Out"=w606:u32, "Image Out"=w597:T1, "Session Out"=w604:T2)  [unwired: 5 in]
            n205 = Bundle By Name(cluster=w605, "IMAQdx Session"=w604) -> (w603:T4)
            n206 = call-poly "IMAQ Extract Tetragon"("Options"=T8 {"Interpolation Type"=enum."Bilinear Fixed", "Destination Width"=0, "Destination Height"=0, "Fill Value"=0.0}, "error in (no error)"=w609, "Tetragon"=w608, "Image Dst"=w600, "Image Src"=w597) -> ("error out"=w595:errorcluster, "Image Dst Out"=w596:T1)  [unwired: 5 in]
            n207 = call <vilib>:"Vision Acquisition CalculateFPS.vi"("buffer number"=w606) -> ("acquired FPS"=w607:dbl)  [unwired: 2 out]
            n208 = local write "Rep. Fps"(w607) -> ()
            n209 = call "IMAQ Rotate"("error in (no error)"=w595, "Angle (degrees)"=sgl 180.0, "Image Dst"=w598, "Image Src"=w596) -> ("error out"=w602:errorcluster, "Image Dst Out"=w601:T1)  [unwired: 6 in]
          }
          frame "PhotonFocus" {
            n210 = Unbundle(w620) -> ("IMAQ Session Out"=w628:refnum<k11>, "OriginalImage"=w627:T1, "error out"=w626:errorcluster, "size"=w625:cluster{dbl, i32}[], "Cropped Image"=w624:T1)  [unwired: 5 out]
            n211 = call <vilib>:"IMAQ Grab Acquire.vi"("error in (no error)"=w626, "Immediate?"=FALSE, "Image In"=w627, "IMAQ Session In"=w628) -> ("error out"=w630:errorcluster, "Acquired Buffer Number"=w629:u32, "Image Out"=w623:T1, "IMAQ Session Out"=w619:refnum<k11>)  [unwired: 4 out]
            n212 = Bundle By Name(cluster=w620, "IMAQ Session Out"=w619) -> (w617:T4)
            n213 = call-poly "IMAQ Extract Tetragon"("error in (no error)"=w630, "Tetragon"=w625, "Image Dst"=w624, "Image Src"=w623) -> ("error out"=w614:errorcluster, "Image Dst Out"=w615:T1)  [unwired: 6 in]
            n214 = call <vilib>:"Vision Acquisition CalculateFPS.vi"("buffer number"=w629) -> ("acquired FPS"=→"Rep. Fps":dbl)  [unwired: 2 out]
            n215 = call "IMAQ Rotate"("error in (no error)"=w614, "Angle (degrees)"=sgl 180.0, "Image Src"=w615) -> ("error out"=w616:errorcluster, "Image Dst Out"=w618:T1)  [unwired: 7 in]
          }
        }
        "Frames" <- w560
        n216 = Divide(x=w574, y=1000.0) -> (x/y=w573:dbl)
        n217 = Divide(x=u32 1000, y=w579) -> (x/y=w571:dbl)
        "Fps" <- w571
        n218 = Round To Nearest(number=w573) -> (nearest integer value=→"Rec Time":dbl)
        n219 = Insert Into Array(array=w570, new element=w571) -> (w569:dbl[])  [unwired: 1 in]
        n220 = Unbundle By Name(w551) -> ()  [unwired: 1 out]
        n221 = call "IMAQ Resample"("X Resolution"="Final res.", "Y Resolution"="Final res.", "error in (no error)"=w552, "Interpolation Type"=w558, "Image Dst"=w561, "Image Src"=w561) -> ("error out"=w556:errorcluster, "Image Dst Out"=w550:T1)  [unwired: 4 in]
        n222 = call "IMAQ Cast Image"("Image Type"=w548, "Image Dst"=w547, "Image Src"=w550) -> ("Image Dst Out"=w549:T1)  [unwired: 7 in, 1 out]
        n223 = local read "Recording"() -> (w562:bool)
        n224 = Enqueue Element(queue=w557, element=w549, error in (no error)=w556) -> (error out=w555:errorcluster)  [unwired: 1 in, 2 out]
        n225 = local write "Rec"(w562) -> ()
        n226 = call "IMAQ ImageToArray"("error in (no error)"=w555, "Image"=w549) -> ("Image Pixels (U16)"=w546:u16[][], "error out"=w564:errorcluster)  [unwired: 2 in, 3 out]
        n227 = case "write into file" shown="True" w562 {
          tunnel: w564 -> [w632 w635]
          tunnel: w546 -> [_ w636]
          tunnel: [w632 w634] -> w565
          tunnel: w581 -> [_ w633]
          frame False {
          }
          frame True {
            n228 = call-poly <instrlib>:"niHWS Write.vi"("error in (no error)"=w635, "data"=w636, "waveform reference in"=w633) -> ("error out"=w634:errorcluster)  [unwired: 7 in, 1 out]
          }
        }
        n229 = Unbundle By Name(w565) -> ("status"=w563:bool)
        n230 = Or(x=w563, y="stop") -> (x .or. y?=w566:bool)
        "Numeric" <- w559
      }
      n231 = call <vilib>:"DAQmx Start Task.vi"("task/channels in"=w211) -> ("task out"=w229:refnum<k21>, "error out"=w223:errorcluster)  [unwired: 13 in]
      n232 = while {
        tunnel: w229 -> [w539]
        tunnel: w223 -> [w535]
        tunnel: w226 -> [w538]
        tunnel: [w532] -> w216
        tunnel: [w536] -> w230
        stop <- w528 stop-if-true
        n233 = local read "Recording"() -> (w533:bool)
        n234 = call-poly <vilib>:"DAQmx Read.vi"("task/channels in"=w539, "timeout"=-1.0, "error in"=w535) -> ("task out"=w536:refnum<k21>, "data"=w537:waveform(dbl), "error out"=w531:errorcluster)  [unwired: 10 in]
        "Photodiode display" <- w537
        n235 = case shown="True" w533 {
          tunnel: w537 -> [_ w542]
          tunnel: w538 -> [_ w545]
          tunnel: [w541 w544] -> w532
          tunnel: w531 -> [w541 w543]
          frame False {
          }
          frame True {
            n236 = call-poly <instrlib>:"niHWS Write.vi"("error in (no error)"=w543, "analog waveform"=w542, "waveform reference in"=w545) -> ("error out"=w544:errorcluster)  [unwired: 7 in, 1 out]
          }
        }
        n237 = Unbundle By Name(w532) -> ("status"=w529:bool)
        n238 = local read "stop"() -> (w534:bool)
        n239 = Or(x=w529, y=w534) -> (x .or. y?=w528:bool)
        n240 = case shown="True" w528 {
          selector: w528 -> [_ w540]
          frame False {
          }
          frame True {
            n241 = local write "stop"(w540) -> ()
          }
        }
      }
      n242 = Unbundle By Name(w198) -> ("Camera"=w199:string)
      n243 = case shown="\"Dalsa Nano\"" w199 {
        tunnel: [w232 w238 w243] -> w219
        tunnel: w215 -> [w233 w239 w242]
        tunnel: w198 -> [w235 w237 w241]
        frame "Dalsa", Default {
          n244 = Unbundle By Name(w235) -> ("IMAQ Session Out"=w234:refnum<k11>)
          n245 = call <vilib>:"IMAQ Close.vi"("error in (no error)"=w233, "IMAQ Session In"=w234) -> ("error out"=w232:errorcluster)  [unwired: 9 out]
        }
        frame "Dalsa Nano" {
          n246 = Unbundle By Name(w237) -> ("IMAQdx Session"=w236:T2)
          n247 = call <vilib>:"IMAQdx Close Camera.vi"("error in"=w239, "Session In"=w236) -> ("error out"=w238:errorcluster)  [unwired: 9 in]
        }
        frame "PhotonFocus" {
          n248 = Unbundle By Name(w241) -> ("IMAQ Session Out"=w240:refnum<k11>)
          n249 = call <vilib>:"IMAQ Close.vi"("error in (no error)"=w242, "IMAQ Session In"=w240) -> ("error out"=w243:errorcluster)  [unwired: 9 out]
        }
      }
      n250 = call <vilib>:"DAQmx Stop Task.vi"("task/channels in"=w230, "error in"=w216) -> ("task out"=w227:refnum<k21>, "error out"=w228:errorcluster)  [unwired: 12 in]
      n251 = call <vilib>:"DAQmx Clear Task.vi"("task in"=w227, "error in"=w228) -> ("error out"=w214:errorcluster)  [unwired: 13 in]
      n252 = local read "Recording"() -> (w213:bool)
      n253 = Merge Errors(w207, w219, w214) -> (w218:errorcluster)
      n254 = case shown="True" w213 {
        tunnel: [w478 w493] -> w224
        tunnel: w220 -> [_ w492]
        tunnel: w218 -> [w478 w479]
        tunnel: w217 -> [_ w480]
        frame False {
        }
        frame True {
          n255 = Delete From Array(array=w492, index=0) -> (array with subset deleted=w490:dbl[])  [unwired: 1 in, 1 out]
          n256 = call-poly <vilib>:"Mean.vi"("X"=w490) -> ("mean"=w491:dbl)  [unwired: 1 out]
          n257 = Build Array(w491) -> (w486:dbl[])
          n258 = flat-sequence {
            tunnel: w486 -> [w497]
            tunnel: [w502] -> w488
            tunnel: [w496] -> w487
            tunnel: w479 -> [w495]
            tunnel: w488 -> [w504]
            tunnel: w487 -> [w513]
            tunnel: [w512] -> w485
            tunnel: [w510] -> w483
            tunnel: [w506] -> w481
            tunnel: w480 -> [w503]
            tunnel: w485 -> [w524]
            tunnel: [w523] -> w484
            tunnel: w483 -> [w522]
            tunnel: [w520] -> w482
            tunnel: w481 -> [w517]
            frame #0 {
              n259 = local read "file handle out"() -> (w494:u32)
              n260 = call <instrlib>:"niHWS New Wfm Reference.vi"("error in (no error)"=w495, "waveform name (empty)"="hz" ("group name (empty)"), "group name (empty)"="imaging", "file handle in"=w494) -> ("error out"=w498:errorcluster, "waveform reference"=w499:u32, "file handle out"=w496:u32)  [unwired: 5 in]
              n261 = call-poly <instrlib>:"niHWS Write.vi"("error in (no error)"=w498, "data"=w497, "waveform reference in"=w499) -> ("error out"=w502:errorcluster)  [unwired: 7 in, 1 out]
            }
            frame #1 {
              n262 = call "IMAQ GetImageSize"("Image"=w503, "error in (no error)"=w504) -> ("Y Resolution"=w506:i32, "X Resolution"=w507:i32, "error out"=w505:errorcluster)  [unwired: 2 in]
              n263 = To Double Precision Float(number=w507) -> (double precision float=w508:dbl)
              n264 = Build Array(w508) -> (w509:dbl[])
              n265 = call <instrlib>:"niHWS New Wfm Reference.vi"("error in (no error)"=w505, "waveform name (empty)"="x" ("group name (empty)"), "group name (empty)"="imaging", "file handle in"=w513) -> ("error out"=w511:errorcluster, "waveform reference"=w514:u32, "file handle out"=w512:u32)  [unwired: 5 in]
              n266 = call-poly <instrlib>:"niHWS Write.vi"("error in (no error)"=w511, "data"=w509, "waveform reference in"=w514) -> ("error out"=w510:errorcluster)  [unwired: 7 in, 1 out]
            }
            frame #2 {
              n267 = To Double Precision Float(number=w517) -> (double precision float=w518:dbl)
              n268 = Build Array(w518) -> (w519:dbl[])
              n269 = call <instrlib>:"niHWS New Wfm Reference.vi"("error in (no error)"=w522, "waveform name (empty)"="y" ("group name (empty)"), "group name (empty)"="imaging", "file handle in"=w524) -> ("error out"=w521:errorcluster, "waveform reference"=w527:u32, "file handle out"=w523:u32)  [unwired: 5 in]
              n270 = call-poly <instrlib>:"niHWS Write.vi"("error in (no error)"=w521, "data"=w519, "waveform reference in"=w527) -> ("error out"=w520:errorcluster)  [unwired: 7 in, 1 out]
            }
          }
          n271 = call <instrlib>:"niHWS Close File.vi"("error in (no error)"=w482, "file handle"=w484) -> ("error out"=w493:errorcluster)  [unwired: 9 in]
        }
      }
    }
    frame #3 {
      w638 = T11 3 items=["no dialog", "OK message", "continue or stop message", "OK message + warnings", "continue/stop + warnings"] ("type of dialog (OK msg:1)")
      n272 = invoke on="Recording Path" class="Path" method="Reinit To Default"() -> ()  [unwired: 3 in, 3 out]
      n273 = call <vilib>:"General Error Handler.vi"("type of dialog (OK msg:1)"=w638, "error in (no error)"=w637) -> ()  [unwired: 9 in, 5 out]
    }
  }
